vi "ROI entry-Get Zoom setting.vi"(11 "error in (no error)":errorcluster) -> (1 "Frame Size":dbl, 3 "Zoom control ref":refnum<vi>, 4 "Zoom Value":dbl, 6 "POI dwell time":dbl, 8 "AOLZ Settings":T1, 10 "Rel. Resolution":dbl, 12 "FOV":dbl, 14 "Laser Power":dbl, 15 "error out":errorcluster)   [LabVIEW 2020]
uses:
  ROI Entry screen/Typedefs/ROI Z-stack settings info.ctl
  ROI Entry screen/Globals/gl_ROI Entry UI globals.vi
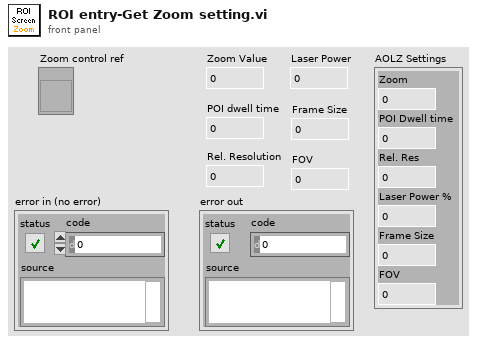
[diagram p1: front panel]
types:
  T1 = typedef "ROI Z-stack settings info.ctl" = cluster{"Zoom":dbl, "POI Dwell time":dbl, "Rel. Res":dbl, "Laser Power %":dbl, "Frame Size":dbl, "FOV":dbl}
  T2 = typedef "ROI entry screen ctrl refs cluster.ctl" = cluster{"Done button":refnum<vi>, "Imaging button":refnum<vi>, "Acquisition button":refnum<vi>, "Scan dwell time per pixel (us)":refnum<vi>, "# of planes":refnum<vi>, "Zoom Ctrl":refnum<vi>, "Equal size":refnum<vi>, "Channel":refnum<vi>, "Image Display":refnum<vi>, "Z-Plane Selector":refnum<vi>, "Number of lines left":refnum<vi>, "Z-stack folder path":refnum<vi>, "POI Density":refnum<vi>, "Arb Plane Entry":refnum<vi>, "Whole Plane":refnum<vi>, "Line Mode":refnum<vi>, "Clear Last":refnum<vi>, "Clear All":refnum<vi>, "Delete Lines":refnum<vi>, "Trial Length (sec)":refnum<vi>, "Palette Type":refnum<vi>, "Intensity slider":refnum<vi>, "# POI":refnum<vi>, "Max Z Proj":refnum<vi>, "Zplane ind":refnum<vi>, "Wavelength (nm)":refnum<vi>, "Number of Trials":refnum<vi>, "Funct stim.trig.enable":refnum<vi>, "Funct stim.trig.delay (s)":refnum<vi>, "Line Mode":refnum<vi>, "Step size (µm)":refnum<vi>, "ROI move mode":refnum<vi>, "Cool-down time (s)":refnum<vi>, "Enable cool-down time":refnum<vi>, "Motor Z ind. (um)":refnum<vi>, "AOL Z ind. (um)":refnum<vi>, "Load Reference Image":refnum<vi>, "Rel.  Res.":refnum<vi>, "ROI LIST":refnum<vi>, "Show All":refnum<vi>, "ROI Type":refnum<vi>, "Start Plane":refnum<vi>, "Stop Plane":refnum<vi>, "Offset ROI":refnum<vi>, "Tab Control":refnum<vi>, "Laser Power(%)":refnum<vi>, "Cycle rate":refnum<vi>, "FOV (Ind.)":refnum<vi>, "Frame Size (Ind.)":refnum<vi>, "Resolution (Ind.)":refnum<vi>, "Pixel Density (Ind)":refnum<vi>, "Laser Power (Ind.)":refnum<vi>, "Dwell Time (Ind.)":refnum<vi>, "Adj MC":refnum<vi>}
  T3 = cluster{"Value":dbl, "Value":dbl, "Value":dbl, "Value":dbl, "Value":dbl, "Value":dbl}
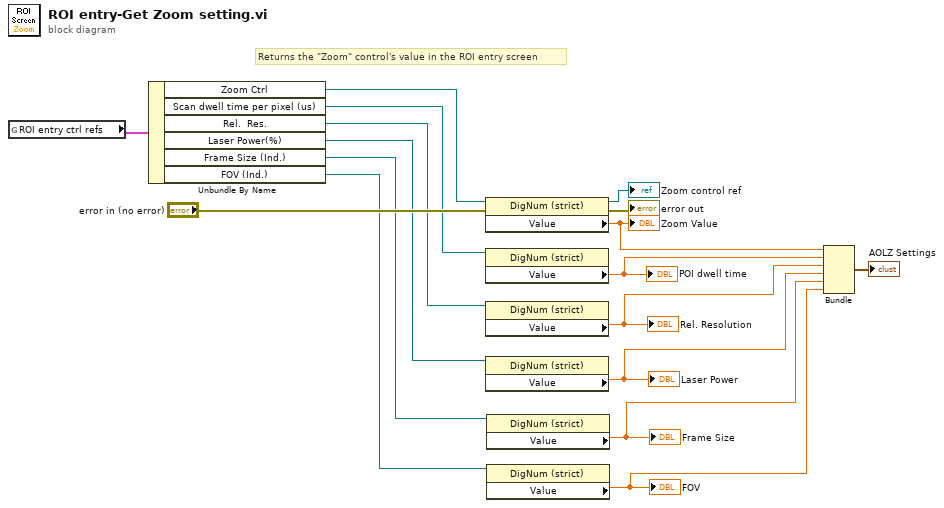
[diagram p0: block diagram]
diagram:
  # "Returns the \"Zoom\" control's value in the ROI entry screen"
  n1 = global read "gl_ROI Entry UI globals.vi" "ROI entry ctrl refs"() -> (w14:T2)
  n2 = Unbundle By Name(w14) -> ("Zoom Ctrl"=w15:refnum<vi>, "Scan dwell time per pixel (us)"=w12:refnum<vi>, "Rel.  Res."=w11:refnum<vi>, "Laser Power(%)"=w10:refnum<vi>, "Frame Size (Ind.)"=w9:refnum<vi>, "FOV (Ind.)"=w8:refnum<vi>)
  n3 = property on="Property Node" class="DigNum (strict)"(reference=w15, error in="error in (no error)") -> (reference out=→"Zoom control ref":refnum<vi>, error out=→"error out":errorcluster, "Value"=w7:dbl)
  "Zoom Value" <- w7
  n4 = property on="Property Node" class="DigNum (strict)"(reference=w12) -> ("Value"=w6:dbl)  [unwired: 1 in, 2 out]
  "POI dwell time" <- w6
  n5 = property on="Property Node" class="DigNum (strict)"(reference=w11) -> ("Value"=w5:dbl)  [unwired: 1 in, 2 out]
  "Rel. Resolution" <- w5
  n6 = property on="Property Node" class="DigNum (strict)"(reference=w10) -> ("Value"=w4:dbl)  [unwired: 1 in, 2 out]
  "Laser Power" <- w4
  n7 = property on="Property Node" class="DigNum (strict)"(reference=w9) -> ("Value"=w3:dbl)  [unwired: 1 in, 2 out]
  "Frame Size" <- w3
  n8 = property on="Property Node" class="DigNum (strict)"(reference=w8) -> ("Value"=w2:dbl)  [unwired: 1 in, 2 out]
  "FOV" <- w2
  n9 = Bundle("Value"=w7, "Value"=w6, "Value"=w5, "Value"=w4, "Value"=w3, "Value"=w2) -> (→"AOLZ Settings":T3)  [unwired: 1 in]
